vi "MakePosCommand.vi"(7 "MxID":u8=254 format="%x", 8 "error in":errorcluster, 10 "Param":u16=4095, 11 "RegAddr":u8=6 format="%x") -> (0 "error out":errorcluster, 3 "Data":u8[](array[numeric]))   [LabVIEW 2014]
panel:
  out "Sum":u8
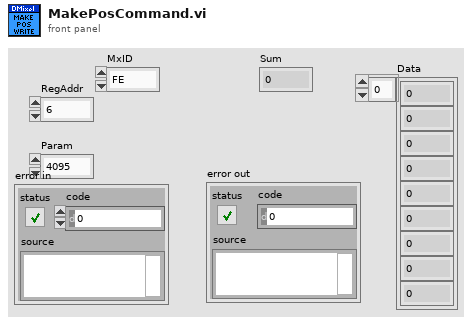
[diagram p1: front panel]
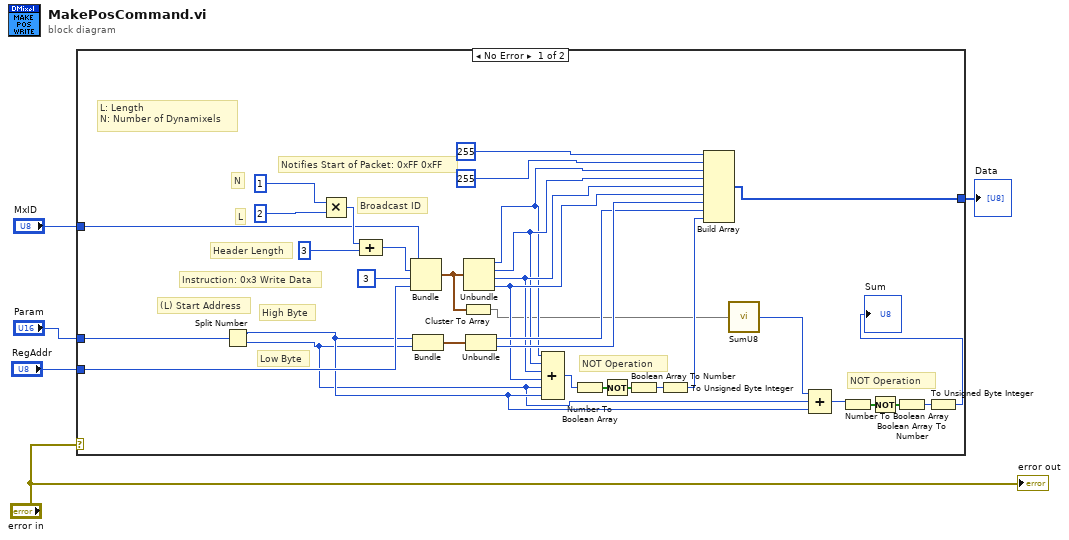
[diagram p0: block diagram]
diagram:
  n1 = case shown="No Error" "error in" {
    tunnel: "RegAddr" -> [w28 _]
    tunnel: "Param" -> [w6 _]
    tunnel: [w17 _] -> w1
    tunnel: "MxID" -> [w18 _]
    frame No Error {
      # "NOT Operation"
      # "L"
      # "Low Byte"
      # "High Byte"
      # "NOT Operation"
      # "L: Length \nN: Number of Dynamixels"
      # "Header Length"
      # "N"
      # "(L) Start Address"
      # "Instruction: 0x3 Write Data"
      # "Broadcast ID"
      # "Notifies Start of Packet: 0xFF 0xFF"
      n2 = Split Number(x=w6) -> (hi(x)=w8:u8, lo(x)=w7:u8)
      n3 = Multiply(x=u8 1 ("N"), y=u8 2) -> (x*y=w39:u8)
      n4 = Compound Arithmetic op=unknown(w39, u8 3 ("value")) -> (w38:u8)
      n5 = Bundle("MxID"=w18, w38, u8 3, "RegAddr"=w28) -> (w16:cluster{"MxID":u8, u8, u8, "RegAddr":u8})  [unwired: 1 in]
      n6 = Bundle(w8, w7) -> (w30:cluster{u8, u8})  [unwired: 1 in]
      n7 = Cluster To Array(cluster=w16) -> (array=w15:u8[])
      n8 = Unbundle(w16) -> ("MxID"=w19:u8, w20:u8, w21:u8, "RegAddr"=w22:u8)
      n9 = Unbundle(w30) -> (w23:u8, w24:u8)
      n10 = Compound Arithmetic op=ADD(w19, w20, w21, w22, w7, w8) -> (w31:u8)
      n11 = Number To Boolean Array(number=w31) -> (Boolean array=w32:bool[])
      n12 = Not(x=w32) -> (.not. x?=w33:bool[])
      n13 = Boolean Array To Number(Boolean array=w33) -> (number=w34:u8)
      n14 = To Unsigned Byte Integer(number=w34) -> (unsigned 8bit integer=w25:u8)
      n15 = Build Array(u8 255, u8 255, w19, w20, w21, w22, w24, w23, w25) -> (w17:u8[])
      n16 = call "SumU8.vi"("Array"=w15) -> ("Sum"=w14:u8)
      n17 = Compound Arithmetic op=ADD(w14, w7, w8) -> (w10:u8)
      n18 = Number To Boolean Array(number=w10) -> (Boolean array=w13:bool[])
      n19 = Not(x=w13) -> (.not. x?=w12:bool[])
      n20 = Boolean Array To Number(Boolean array=w12) -> (number=w11:u8)
      n21 = To Unsigned Byte Integer(number=w11) -> (unsigned 8bit integer=→"Sum":u8)
    }
    frame Error {
    }
  }
  "Data" <- w1
  "error out" <- "error in"
